vi "Configure_SL.vi"() -> (1 "changed?":bool, 2 "Property":string[](array[string]))   [LabVIEW 2019]
uses:
  <vilib>/Utility/miscctls.llb/LVRowAndColumnUnsignedTypeDef.ctl
panel:
  out "Table Control":string[][](table)
  out "error out":errorcluster
  in  "Properties":i32(listbox)
  in  "Cancel":bool
  in  "OK":bool
  # "SystemLink Panel\n\nhttps://www.systemlinkcloud.com\n\nAPI: https://api.systemlinkcloud.com"
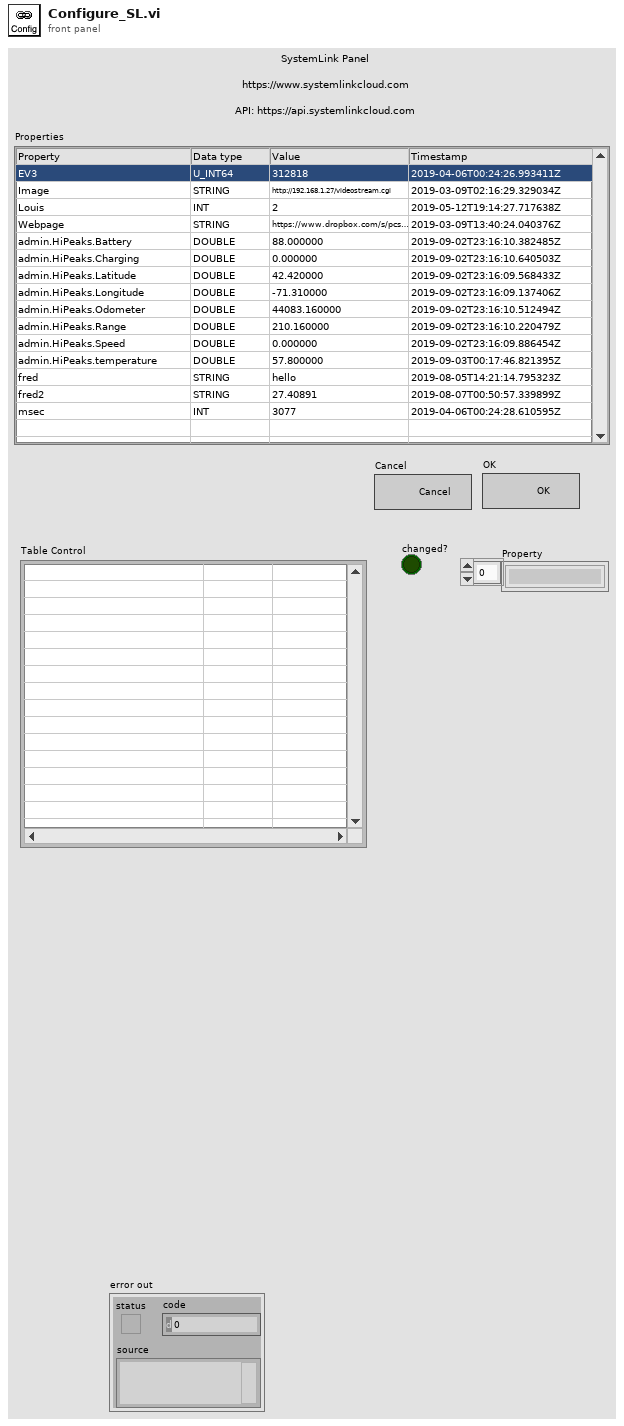
[diagram p1: front panel]
types:
  T1 = enum16{"GET", "PUT", "POST", "MultiPOST", "DELETE"}
  T2 = cluster{"tagsWithValues":cluster{"tag":cluster{"path":string, "type":string}, "current":cluster{"timestamp":string, "value":cluster{"type":string, "value":string}}}[]}
  T3 = typedef "LVRowAndColumnUnsignedTypeDef.ctl" = cluster{"Row":u32, "Column":u32}
  T4 = cluster{"Name":string, "BaseURL":string, "AppKey":string, "Headers":string[], "Timeout":i32}
  T5 = cluster{"url":string, "sent headers":string, "sent body":string, "headers":string, "body":string, "Sent":string, "Received":string}
  T6 = cluster{"tag":cluster{"path":string, "type":string}, "current":cluster{"timestamp":string, "value":cluster{"type":string, "value":string}}}[]
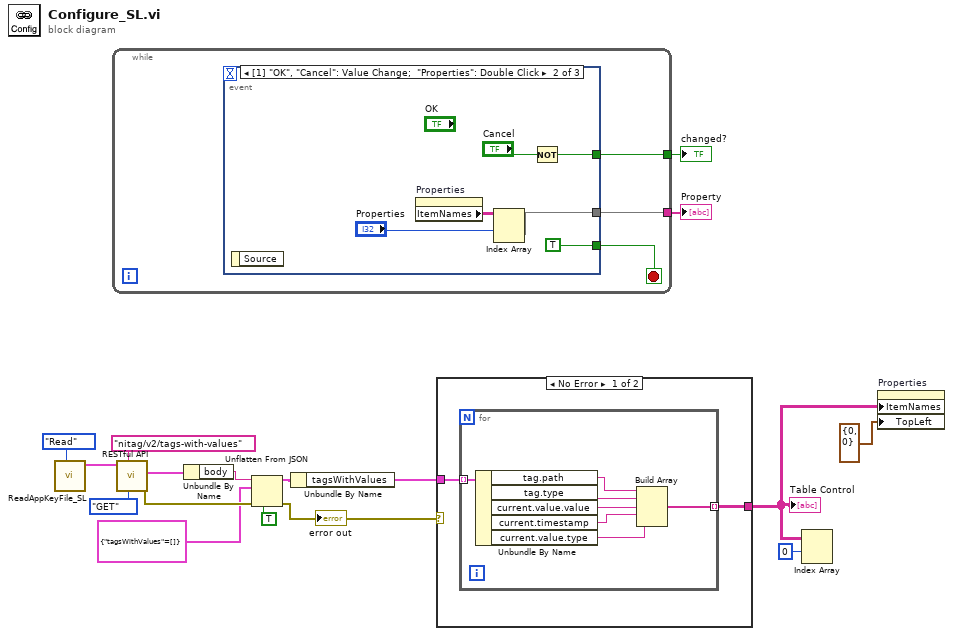
[diagram p0: block diagram]
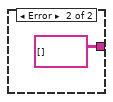
[diagram p2: hidden frame]
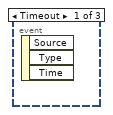
[diagram p3: hidden frame]
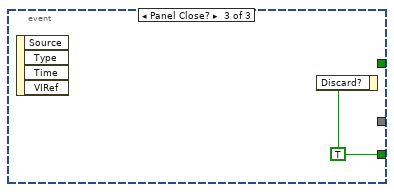
[diagram p4: hidden frame]
diagram:
  n1 = call "ReadAppKeyFile_SL.vi"("Task"=enum16{"Read", "Write"}."Read") -> ("Device Out"=w7:T4)  [unwired: 8 in, 2 out]
  n2 = while {
    tunnel: [w20] -> w17
    tunnel: [w18] -> w16
    stop <- w19 stop-if-true
    n3 = event shown="[1] \"OK\", \"Cancel\": Value Change;  \"Properties\": Double Click" {
      selector: _ -> [_ _ _]
      dyn-events: _ -> [_ _ _]
      timeout: _ -> [_ _ _]
      tunnel: [_ w21 _] -> w20
      tunnel: [_ TRUE w27] -> w19
      tunnel: [_ w23 _] -> w18
      event Timeout {
        n4 = event-data() -> ()  [unwired: 1 in, 3 out]
      }
      event "OK", "Cancel": Value Change; "Properties": Double Click {
        n5 = event-data() -> ()  [unwired: 1 in, 1 out]
        n6 = property on="Properties" class="MCListbox (strict)"() -> ("ItemNames"=w25:string[][])  [unwired: 2 in, 2 out]
        n7 = Index Array(array=w25, index (row)="Properties") -> (element=w23:string[])  [unwired: 1 in]
        n8 = Not(x="Cancel") -> (.not. x?=w21:bool)
      }
      event Panel Close? {
        w27 = TRUE
        n9 = event-data() -> ()  [unwired: 1 in, 4 out]
        n10 = event-data("Discard?"=w27) -> ()  [unwired: 1 in, 1 out]
      }
    }
  }
  "changed?" <- w17
  "Property" <- w16
  n11 = call "RESTful API.vi"("Method"=T1."GET", "url"="nitag/v2/tags-with-values", "Device In"=w7) -> ("error out"=w4:errorcluster, "Comm"=w5:T5)  [unwired: 6 in, 1 out]
  n12 = Unbundle By Name(w5) -> ("body"=w11:string)
  n13 = Unflatten From JSON(JSON string=w11, type and defaults=T2 {"tagsWithValues"=[]}, default null elements? (F)=TRUE, error in (no error)=w4) -> (value=w14:T2, error out=w9:errorcluster)  [unwired: 3 in]
  "error out" <- w9
  n14 = Unbundle By Name(w14) -> ("tagsWithValues"=w12:T6)
  n15 = case shown="No Error" w9 {
    tunnel: w12 -> [w29 _]
    tunnel: [w28 string[][] []] -> w2
    frame No Error {
      n16 = for {
        tunnel: w29 -> [w36] mode=indexing
        tunnel: [w31] -> w28 mode=indexing
        n17 = Unbundle By Name(w36) -> ("tag.path"=w30:string, "tag.type"=w35:string, "current.value.value"=w34:string, "current.timestamp"=w33:string, "current.value.type"=w32:string)
        n18 = Build Array(w30, w35, w34, w33, w32) -> (w31:string[])
      }
    }
    frame Error {
    }
  }
  "Table Control" <- w2
  n19 = Index Array(array=w2, index (row)=0) -> ()  [unwired: 1 in, 1 out]
  n20 = property on="Properties" class="MCListbox (strict)"("ItemNames"=w2, "TopLeft"=T3 {"Row"=0, "Column"=0} ("Top Left Visible Cell")) -> ()  [unwired: 2 in, 2 out]
